vi "ERIO WIN Process Signal Captures.vi"(6 "Supervisory Variables In":T6={"Alarm Threshold"=0.0, "Shutdown"=FALSE, "Enable SNS Alarm"=FALSE, "Enable SNS Stage Notification"=FALSE, "Enable SQS Notification"=FALSE, "Enable S3 TDMS Signal Capture"=FALSE, "Enable SystemLink Signal Capture"=FALSE, "Capture Signal"=FALSE, "Server Update"=FALSE, "AWS Access Key"="AKIAINLDO2Y2PDFEWDOQ", "AWS Secret Key"="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", "Phone Number"="+15037066913", "Region"=enum."us-west-2", "AWS SQS Queue"="+15037066913", "AWS S3 Bucket"="+15037066913"}, 7 "WIN Variables In":T4, 8 "error in (no error)":errorcluster, 9 "AWS Variables In":T8, 10 "Signal Capture File Path":path=path "C:/ERIO Data Files", 11 "EEISysLink.lvclass In":refnum<class "EEISysLink.lvclass">) -> (0 "error out":errorcluster, 1 "AWS Variables Out":T8, 3 "EEISysLink.lvclass Out":refnum<class "EEISysLink.lvclass">, 4 "Supervisory Variables Out":T6={"Alarm Threshold"=0.0, "Shutdown"=FALSE, "Enable SNS Alarm"=FALSE, "Enable SNS Stage Notification"=FALSE, "Enable SQS Notification"=FALSE, "Enable S3 TDMS Signal Capture"=FALSE, "Enable SystemLink Signal Capture"=FALSE, "Capture Signal"=FALSE, "Server Update"=FALSE, "AWS Access Key"="AKIAINLDO2Y2PDFEWDOQ", "AWS Secret Key"="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", "Phone Number"="+15037066913", "Region"=enum."us-west-2", "AWS SQS Queue"="+15037066913", "AWS S3 Bucket"="+15037066913"}, 5 "WIN Variables Out":T4)   [LabVIEW 2017]
doc: "Check for new signal captures from enabled sources and process/display as needed.\n\nJames Tillett P.E.\nEndeavor Engineering Inc.\nwww.endeavoreng.com"
uses:
  Class EEISysLink/EEISysLink.lvclass
  Controls/ERIO AWS Toolkit Variables.ctl
  <vilib>/AWS Toolkit/SQS/Queue/Queue.lvclass
  <vilib>/AWS Toolkit/SNS/Phone Number/Phone Number.lvclass
  <vilib>/AWS Toolkit/S3/Bucket/Bucket.lvclass
  Controls/ERIO Supervisory Variables.ctl
  <vilib>/AWS Toolkit/Core/HTTP Request/Region.ctl
  Controls/ERIO WIN State Variables.ctl
  Controls/ERIO Worker Variables.ctl
  <vilib>/AWS Toolkit/S3/Object Content.ctl
  <vilib>/AWS Toolkit/S3/Storage Class.ctl
  <vilib>/AWS Toolkit/S3/Owner.ctl
  Class EEISysLink/Controls/SL Tag Scope.ctl
  Class EEISysLink/Controls/SL Tag Type.ctl
  <vilib>/AWS Toolkit/Core/HTTP Request/HTTP Request.lvclass
  <vilib>/AWS Toolkit/S3/NI_AWS_S3.lvlib
panel:
  out "S3 Objects Found":T1[](array[typedef])
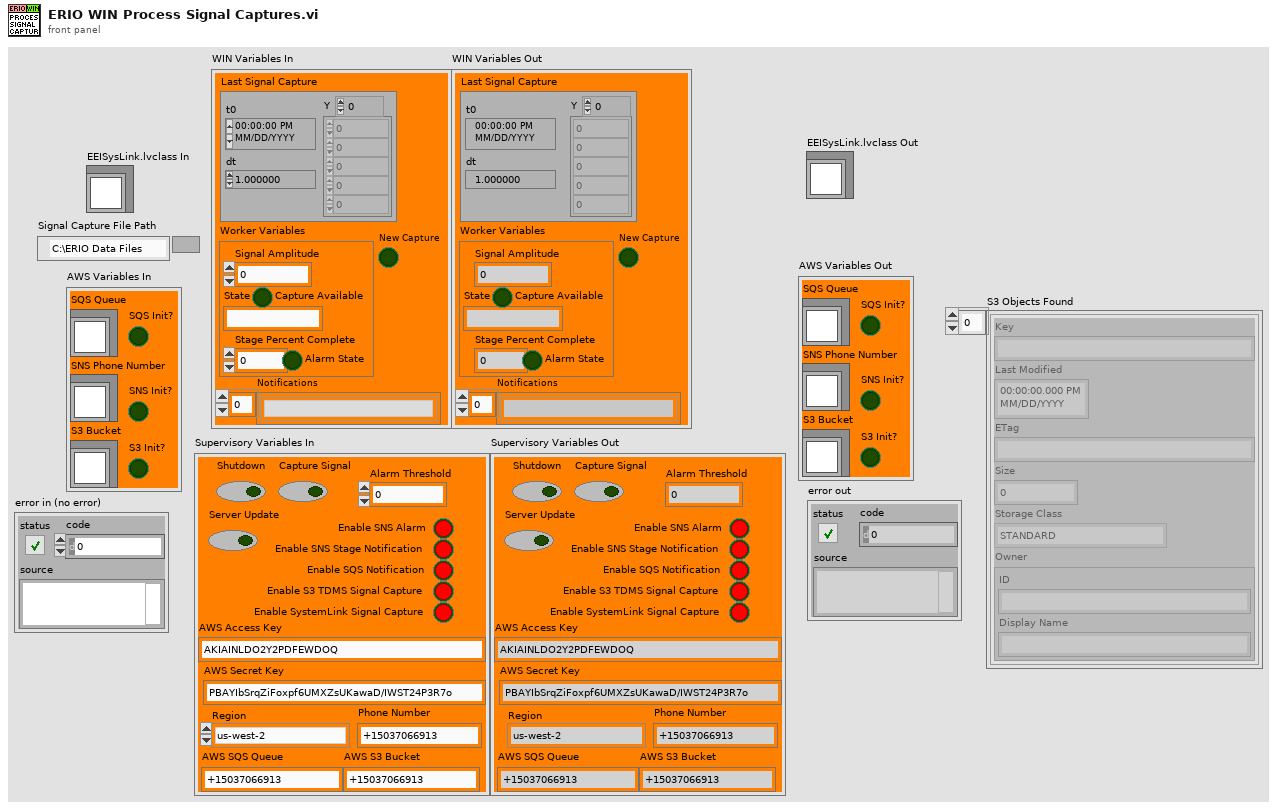
[diagram p1: front panel]
types:
  T1 = typedef "NI_AWS_S3.lvlib/Object Content.ctl" = cluster{"Key":string, "Last Modified":timestamp, "ETag":string, "Size":u64, "Storage Class":T2, "Owner":T3}
  T2 = typedef "NI_AWS_S3.lvlib/Storage Class.ctl" = enum16{"STANDARD", "REDUCED_REDUNDANCY"}
  T3 = typedef "NI_AWS_S3.lvlib/Owner.ctl" = cluster{"ID":string, "Display Name":string}
  T4 = typedef "ERIO WIN State Variables.ctl" = cluster{"Worker Variables":T5, "Notifications":string[], "New Capture":bool, "Last Signal Capture":waveform(dbl)}
  T5 = typedef "ERIO Worker Variables.ctl" = cluster{"Signal Amplitude":dbl, "State":string, "Stage Percent Complete":dbl, "Alarm State":bool, "Capture Available":bool}
  T6 = typedef "ERIO Supervisory Variables.ctl" = cluster{"Alarm Threshold":dbl, "Shutdown":bool, "Enable SNS Alarm":bool, "Enable SNS Stage Notification":bool, "Enable SQS Notification":bool, "Enable S3 TDMS Signal Capture":bool, "Enable SystemLink Signal Capture":bool, "Capture Signal":bool, "Server Update":bool, "AWS Access Key":string, "AWS Secret Key":string, "Phone Number":string, "Region":T7, "AWS SQS Queue":string, "AWS S3 Bucket":string}
  T7 = typedef "NI_AWS_Core.lvlib/HTTP Request.lvclass/Region.ctl" = enum16{"us-east-1", "us-east-2", "us-west-1", "us-west-2", "ap-northeast-1", "ap-northeast-2", "ap-southeast-1", "ap-southeast-2", "ca-central-1", "eu-central-1", "eu-west-1", "eu-west-2", "sa-east-1"}
  T8 = typedef "ERIO AWS Toolkit Variables.ctl" = cluster{"SQS Queue":refnum<class "Queue.lvclass">, "SNS Phone Number":refnum<class "Phone Number.lvclass">, "S3 Bucket":refnum<class "Bucket.lvclass">, "SQS Init?":bool, "S3 Init?":bool, "SNS Init?":bool}
  T9 = typedef "EEISysLink.lvclass/SL Tag Type.ctl" = enum16{"All", "Supervisor", "Worker"}
  T10 = typedef "EEISysLink.lvclass/SL Tag Scope.ctl" = enum16{"Local", "Server"}
  T11 = typedef "SL Tag Value.ctl" = cluster{"Value":variant, "Time Stamp":timestamp, "Tag Data Type":T12, "Name":string}
  T12 = typedef "EEISysLink.lvclass/SL Tag Data Type.ctl" = enum16{"Double", "Integer", "String", "Boolean", "Waveform"}
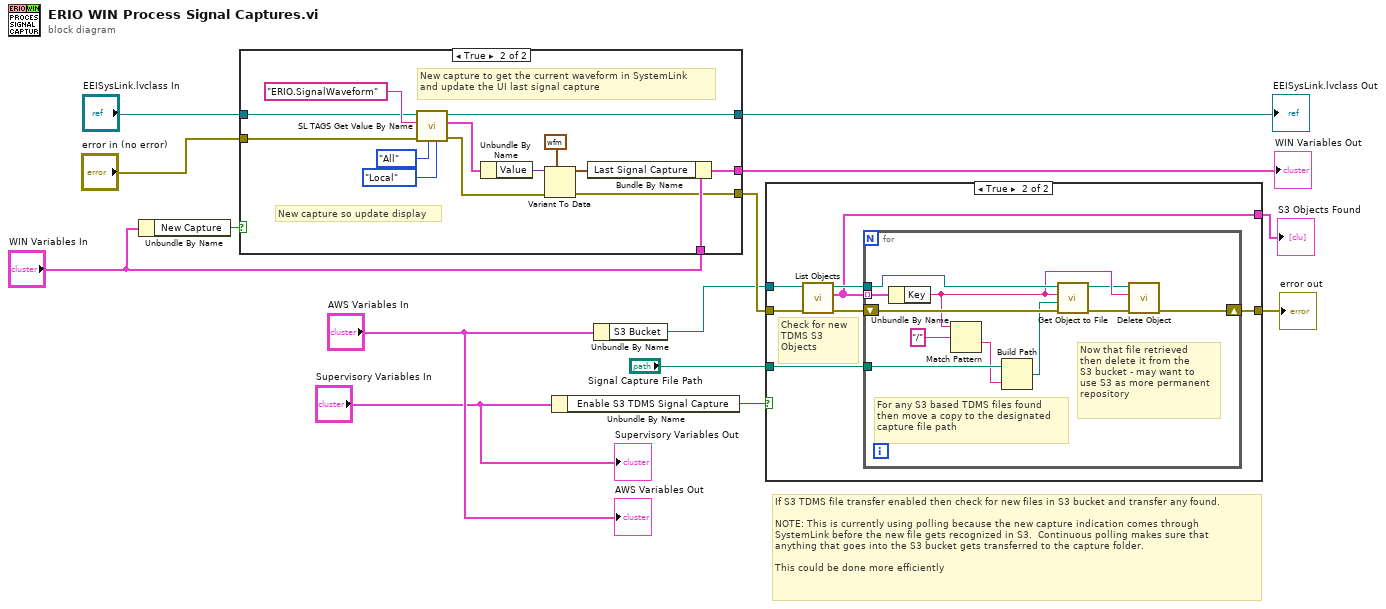
[diagram p0: block diagram]
diagram:
  # "If S3 TDMS file transfer enabled then check for new files in S3 bucket and transfer any found.\n\nNOTE: This is currently using polling because the new capture indication comes through \nSystemLink before the new file gets recognized in S3.  Continuous polling makes sure that\nanything that goes into the S3 bucket gets transferred to the capture folder.  \n\nThis could be done more efficiently"
  n1 = Unbundle By Name("WIN Variables In") -> ("New Capture"=w1:bool)
  n2 = case shown="True" w1 {
    tunnel: [w16 w31] -> w14
    tunnel: "WIN Variables In" -> [w16 w30]
    tunnel: "EEISysLink.lvclass In" -> [w17 w26]
    tunnel: "error in (no error)" -> [w15 w25]
    tunnel: [w17 w21] -> w10
    tunnel: [w15 w18] -> w5
    frame False {
    }
    frame True {
      # "New capture to get the current waveform in SystemLink\nand update the UI last signal capture"
      # "New capture so update display"
      n3 = call-dynamic "SL TAGS Get Value By Name.vi"("Tag Scope"=SL_Tag_Scope."Local", "Tag Type"=SL_Tag_Type."All", "error in (no error)"=w25, "Tag Name"="ERIO.SignalWaveform", "EEISysLink in"=w26) -> ("error out"=w22:errorcluster, "Tag Value"=w23:T11, "EEISysLink out"=w21:refnum<class "EEISysLink.lvclass">)  [unwired: 3 in, 1 out]
      n4 = Unbundle By Name(w23) -> ("Value"=w24:variant)
      n5 = Variant To Data(error in=w22, type=waveform(dbl) {"t0"=timestamp(0 s since 1904-01-01), "dt"=1.0, "Y"=[]} ("waveform in"), Variant=w24) -> (data=w19:waveform(dbl), error out=w18:errorcluster)
      n6 = Bundle By Name(cluster=w30, "Last Signal Capture"=w19) -> (w31:T4)
    }
  }
  "EEISysLink.lvclass Out" <- w10
  "WIN Variables Out" <- w14
  n7 = Unbundle By Name("Supervisory Variables In") -> ("Enable S3 TDMS Signal Capture"=w6:bool)
  n8 = Unbundle By Name("AWS Variables In") -> ("S3 Bucket"=w4:refnum<class "Bucket.lvclass">)
  n9 = case shown="True" w6 {
    tunnel: w4 -> [_ w39]
    tunnel: w5 -> [w32 w38]
    tunnel: [w32 w34] -> w2
    tunnel: "Signal Capture File Path" -> [_ w35]
    tunnel: [_ w33] -> w3
    frame False {
    }
    frame True {
      # "Check for new\nTDMS S3\nObjects"
      n10 = call <vilib>:"List Objects.vi"("error in (no error)"=w38, "Bucket in"=w39) -> ("error out"=w37:errorcluster, "Objects"=w33:T1[], "Bucket out"=w36:refnum<class "Bucket.lvclass">)  [unwired: 6 in, 1 out]
      n11 = for {
        tunnel: w33 -> [w50] mode=indexing
        shift-right: [w40] -> w34
        shift-left: w37 -> [w48]
        tunnel: w36 -> [w49]
        tunnel: w35 -> [w46]
        # "Now that file retrieved\nthen delete it from the\nS3 bucket - may want to\nuse S3 as more permanent\nrepository"
        # "For any S3 based TDMS files found\nthen move a copy to the designated\ncapture file path"
        n12 = Unbundle By Name(w50) -> ("Key"=w42:string)
        n13 = Match Pattern(string=w42, regular expression="/") -> (after substring=w45:string)  [unwired: 1 in, 3 out]
        n14 = Build Path(base path=w46, name or relative path=w45) -> (appended path=w44:path)
        n15 = call <vilib>:"Get Object to File.vi"("error in (no error)"=w48, "File"=w44, "Object Path"=w42, "Bucket in"=w49) -> ("error out"=w43:errorcluster, "Bucket out"=w41:refnum<class "Bucket.lvclass">)  [unwired: 6 in]
        n16 = call <vilib>:"Delete Object.vi"("error in (no error)"=w43, "Object Key"=w42, "Bucket in"=w41) -> ("error out"=w40:errorcluster)  [unwired: 7 in, 1 out]
      }
    }
  }
  "error out" <- w2
  "S3 Objects Found" <- w3
  "AWS Variables Out" <- "AWS Variables In"
  "Supervisory Variables Out" <- "Supervisory Variables In"
